vi "tcp_send_packet.vi"(8 "error in (no error)":errorcluster, 10 "tcp_packet":T1, 11 "TCP Network Connection in":refnum<k5>) -> (0 "error out":errorcluster, 3 "TCP Network Connection out":refnum<k5>)   [LabVIEW 2021]
uses:
  typedefs/tcp_packet.ctl
  typedefs/tcp_cmd.ctl
  typedefs/tcp_states.ctl
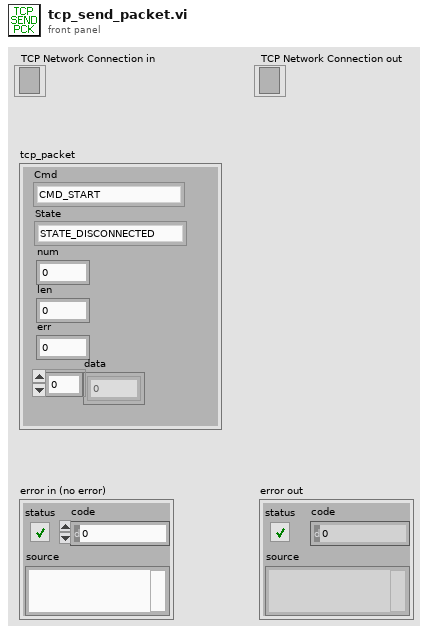
[diagram p1: front panel]
types:
  T1 = typedef "tcp_packet.ctl" = cluster{"Cmd":T2, "State":T3, "num":u32, "len":u32, "err":u32, "data":u32[]}
  T2 = typedef "tcp_cmd.ctl" = enum32{"CMD_START", "CMD_SOFTTRIG", "CMD_SETTSET", "CMD_SETTREAD", "CMD_TRANS_START", "CMD_TRANS_LEN", "CMD_TRANS_FINISH"}
  T3 = typedef "tcp_states.ctl" = enum32{"STATE_DISCONNECTED", "STATE_IDLE", "STAIT_WAITINGTRIG", "STATE_ACQUISITION", "STATE_DATARDY", "STATE_DATATRANS", "STATE_ERROR"}
  T4 = enum16{"big-endian, network order", "native, host order", "little-endian"}
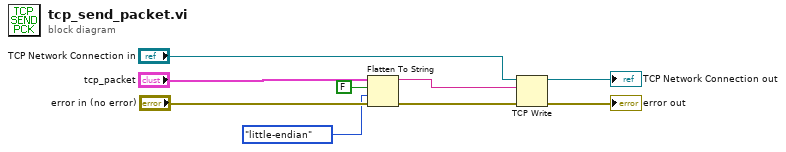
[diagram p0: block diagram]
diagram:
  n1 = Flatten To String(anything="tcp_packet", prepend array or string size? (T)=FALSE, byte order (0:big-endian, network order)=T4."little-endian", error in (no error)="error in (no error)") -> (data string=w4:string, error out=w3:errorcluster)  [unwired: 1 out]
  n2 = TCP Write(connection ID="TCP Network Connection in", data in=w4, error in (no error)=w3) -> (connection ID out=→"TCP Network Connection out":refnum<k5>, error out=→"error out":errorcluster)  [unwired: 1 in, 1 out]
